vi "test_buttons.vi"() -> ()   [LabVIEW 2018]
panel:
  in  "ValveManualCluster":refnum<vi>
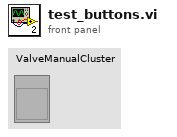
[diagram p1: front panel]
types:
  T1 = cluster{"C8":bool, "C7":bool, "C6":bool, "C5":bool, "C4":bool, "C3":bool, "C2":bool, "C1":bool, "B8":bool, "B7":bool, "B6":bool, "B5":bool, "B4":bool, "B3":bool, "B2":bool, "B1":bool, "A8":bool, "A7":bool, "A6":bool, "A5":bool, "A4":bool, "A3":bool, "A2":bool, "A1":bool}
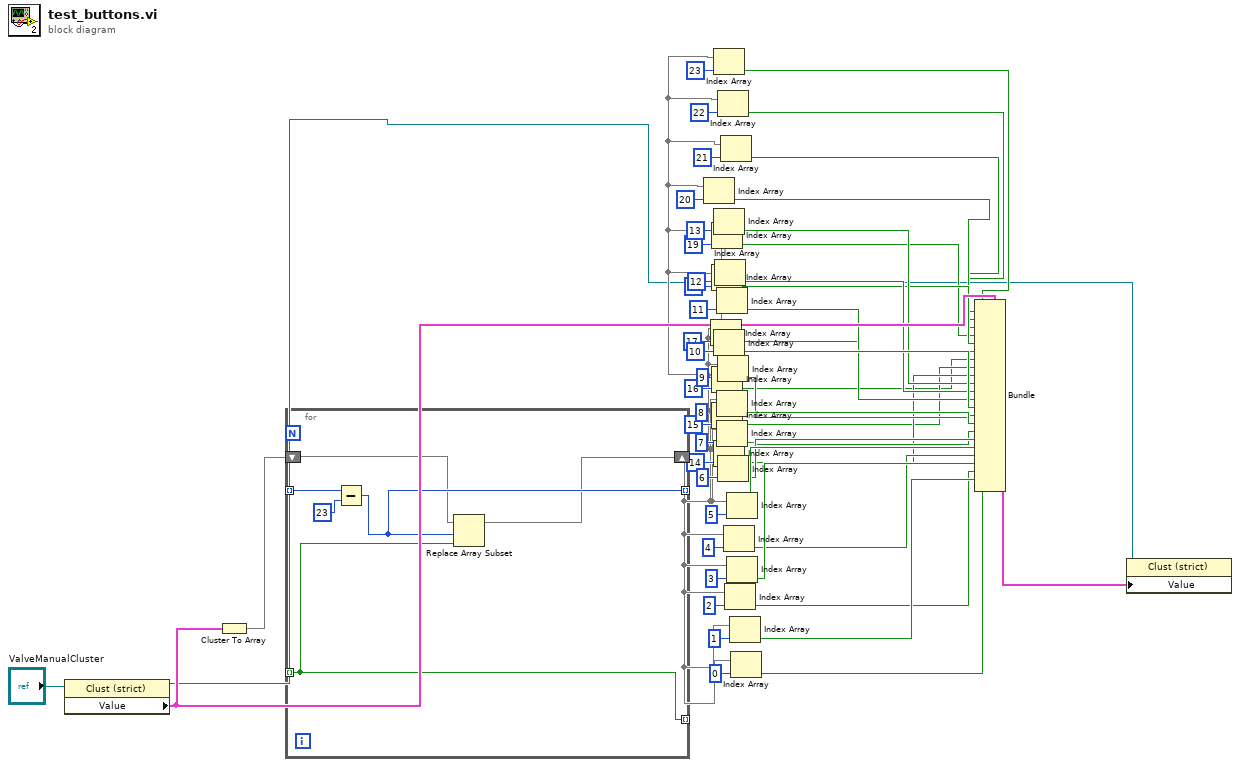
[diagram p0: block diagram]
diagram:
  n1 = property class="Clust (strict)"(reference="ValveManualCluster") -> (reference out=w1:refnum<vi>, "Value"=w52:T1)  [unwired: 1 in, 1 out]
  n2 = Cluster To Array(cluster=w52) -> (array=w53:bool[])
  n3 = for {
    tunnel: _ -> [w60] mode=indexing
    tunnel: [w57] -> _ mode=indexing
    tunnel: _ -> [w58] mode=indexing
    tunnel: [w58] -> _ mode=indexing
    shift-right: [w56] -> w5
    shift-left: w53 -> [w55]
    n4 = Subtract(x=w60, y=23) -> (x-y=w57:i32)
    n5 = Replace Array Subset(array=w55, new element=w58, index=w57) -> (w56:bool[])
  }
  n6 = Index Array(array=w5, index=20) -> (element=w9:bool)
  n7 = Index Array(array=w5, index=17) -> (element=w12:bool)
  n8 = Index Array(array=w5, index=19) -> (element=w10:bool)
  n9 = Index Array(array=w5, index=18) -> (element=w11:bool)
  n10 = Index Array(array=w5, index=16) -> (element=w13:bool)
  n11 = Index Array(array=w5, index=15) -> (element=w19:bool)
  n12 = Index Array(array=w5, index=23) -> (element=w2:bool)
  n13 = Index Array(array=w5, index=13) -> (element=w21:bool)
  n14 = Index Array(array=w5, index=10) -> (element=w24:bool)
  n15 = Index Array(array=w5, index=14) -> (element=w20:bool)
  n16 = Index Array(array=w5, index=12) -> (element=w22:bool)
  n17 = Index Array(array=w5, index=11) -> (element=w23:bool)
  n18 = Index Array(array=w5, index=8) -> (element=w26:bool)
  n19 = Index Array(array=w5, index=7) -> (element=w27:bool)
  n20 = Index Array(array=w5, index=22) -> (element=w3:bool)
  n21 = Index Array(array=w5, index=9) -> (element=w25:bool)
  n22 = Index Array(array=w5, index=6) -> (element=w28:bool)
  n23 = Index Array(array=w5, index=21) -> (element=w4:bool)
  n24 = Index Array(array=w5, index=4) -> (element=w40:bool)
  n25 = Index Array(array=w5, index=2) -> (element=w42:bool)
  n26 = Index Array(array=w5, index=5) -> (element=w39:bool)
  n27 = Index Array(array=w5, index=3) -> (element=w41:bool)
  n28 = Index Array(array=w5, index=1) -> (element=w43:bool)
  n29 = Index Array(array=w5, index=0) -> (element=w51:bool)
  n30 = Bundle(cluster=w52, "C8"=w2, "C7"=w3, "C6"=w4, "C5"=w9, "C4"=w10, "C3"=w11, "C2"=w12, "C1"=w13, "B8"=w19, "B7"=w20, "B6"=w21, "B5"=w22, "B4"=w23, "B3"=w24, "B2"=w25, "B1"=w26, "A8"=w27, "A7"=w28, "A6"=w39, "A5"=w40, "A4"=w41, "A3"=w42, "A2"=w43, "A1"=w51) -> (w49:T1)
  n31 = property class="Clust (strict)"(reference=w1, "Value"=w49) -> ()  [unwired: 1 in, 2 out]
